vi "PWM1.vi"() -> ()   [LabVIEW 2019]
uses:
  <vilib>/rvi/Emulation/niFpgaGetClockAttributes.vi
  <vilib>/rvi/Emulation/niFpgaSctlEmulationGetInTimedLoop.vi
  <vilib>/rvi/Emulation/niFpgaEmulationReportErrorSimple.vi
  <vilib>/rvi/eio/common/nirviEmuTemplateMethod_errors.vi
  <vilib>/rvi/Emulation/niFpgaCriticalErrorInLSC.vi
  <vilib>/eio/EIONode/EIONode.xnode
panel:
  out "x-1":u16
  out "波形图表":u16(graph)
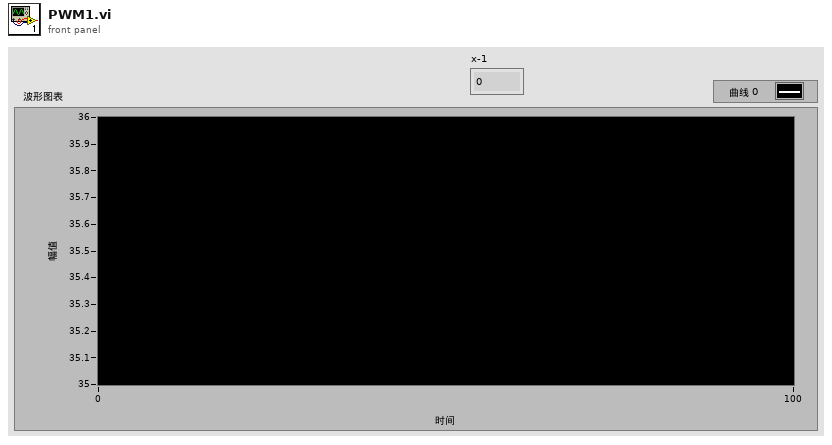
[diagram p1: front panel]
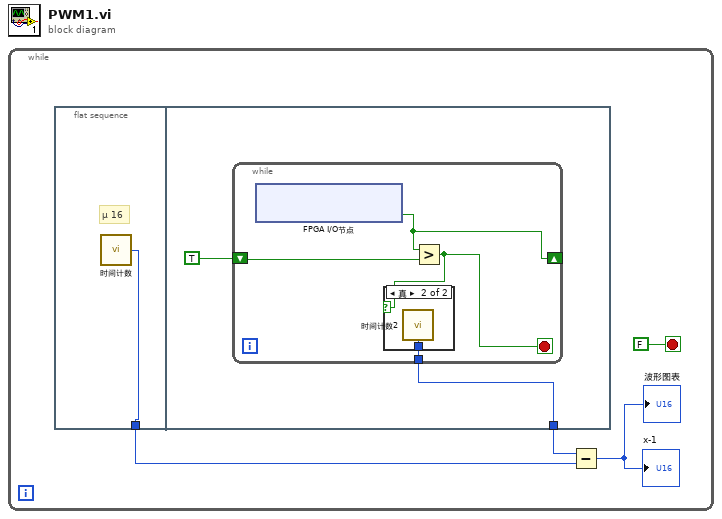
[diagram p0: block diagram]
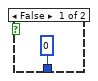
[diagram p2: hidden frame]
diagram:
  n1 = while {
    stop <- FALSE stop-if-true
    n2 = flat-sequence {
      tunnel: [w5] -> w3
      tunnel: [w6] -> w2
      frame #0 {
        # "μ 16"
        n3 = call "时间计数"() -> ("Tick Count(uSec)"=w5:u16)
      }
      frame #1 {
        n4 = while {
          shift-right: [w10] -> _
          shift-left: TRUE -> [w11]
          tunnel: [w8] -> w6
          stop <- w9 stop-if-true
          n5 = xnode "FPGA I/O节点"() -> ("ConnectorB/DIO0"=w10:bool)  [unwired: 1 in, 1 out]
          n6 = Greater?(x=w10, y=w11) -> (0:w9:bool)
          n7 = case shown="真" w9 {
            tunnel: [u16 0 ("Tick Count(uSec)") w13] -> w8
            frame False {
            }
            frame True {
              n8 = call "时间计数2"() -> ("Tick Count(uSec)"=w13:u16)
            }
          }
        }
      }
    }
    n9 = Subtract(x=w2, y=w3) -> (x-y=→"x-1" →"波形图表":u16)
  }
